vi "NI VeriStand - Close Error Message Notification.vi"(8 "error in (no error)":errorcluster, 11 "ErrorMessage Refs":T1) -> (0 "error out":errorcluster)   [LabVIEW 2020, in "NI_VS MacroPlayerAPI.lvlib"]
doc: "Closes an open reference to error messages the Macro Player sends. Use the Open Error Message Notification VI to open the reference this VI closes."
uses:
  <vilib>/NI VeriStand/Execution/MacroPlayer/NI_VS MacroPlayerAPI.lvlib
  <vilib>/NI VeriStand/Execution/MacroPlayer/ErrorMessage Refs.ctl
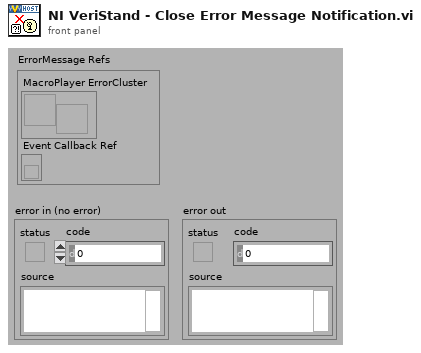
[diagram p1: front panel]
types:
  T1 = typedef "NI_VS MacroPlayerAPI.lvlib/ErrorMessage Refs.ctl" = cluster{"MacroPlayer ErrorCluster":refnum<user-event>, "Event Callback Ref":refnum<k27>}
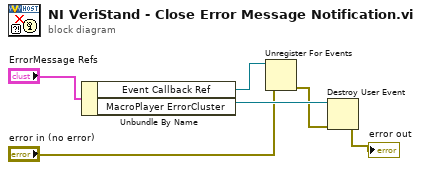
[diagram p0: block diagram]
diagram:
  n1 = Unbundle By Name("ErrorMessage Refs") -> ("Event Callback Ref"=w6:refnum<k27>, "MacroPlayer ErrorCluster"=w5:refnum<user-event>)
  n2 = Unregister For Events(event registration refnum=w6, error in="error in (no error)") -> (error out=w4:errorcluster)
  n3 = Destroy User Event(user event=w5, error in=w4) -> (error out=→"error out":errorcluster)
